vi "CVT2IndexReadTest.vi"() -> (3 "Unit Test Framework Results":T1)   [LabVIEW 2013, in "UnitTests.lvlib"]
uses:
  UnitTests.lvlib
  <vilib>/utf/common/utf_test_result_troll.ctl
  <vilib>/utf/common/utf_test_result.ctl
  <vilib>/utf/common/utf_test_result_failure.ctl
  <vilib>/utf/common/utf_test_comparison_operators.ctl
  <vilib>/utf/common/utf_vi_tag.ctl
  <vilib>/NI/Current Value Table/DataTypes/I32_Read Index.vi
  <vilib>/NI/Current Value Table/Memory Block.vi
  <vilib>/NI/Current Value Table/DataTypes/I32_Memory Block.vi
  <vilib>/utf/NI_UnitTestFramework.lvlib
  <vilib>/NI/Current Value Table/Current Value Table.lvlib
panel:
  out "Value":i32
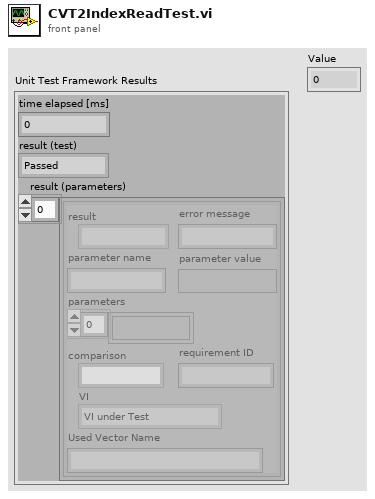
[diagram p1: front panel]
types:
  T1 = typedef "NI_UnitTestFramework.lvlib/utf_test_result_troll.ctl" = cluster{"time elapsed [ms]":u32, "result (test)":T2, "result (parameters)":T3[]}
  T2 = typedef "NI_UnitTestFramework.lvlib/utf_test_result.ctl" = enum16{"Passed", "Failed", "Error", "Skipped", "Not Processed"}
  T3 = typedef "NI_UnitTestFramework.lvlib/utf_test_result_failure.ctl" = cluster{"result":T2, "error message":string, "parameter name":string, "parameter value":variant, "parameters":variant[], "comparison":T4, "requirement ID":string, "VI":T5, "Used Vector Name":string}
  T4 = typedef "NI_UnitTestFramework.lvlib/utf_test_comparison_operators.ctl" = enum16{"=", "!=", ">", ">=", "<", "<=", "range", "symmetric tolerance", "asymmetric tolerance", "string contains", "string not contain", "array size", "string length", "array range", "by element", "array range (limit array)", "user-defined", "array contains", "array not contain", "vector length", "= (elm)", "!= (elm)", "= (case insensitive)", "!= (case insensitive)"}
  T5 = typedef "NI_UnitTestFramework.lvlib/utf_vi_tag.ctl" = enum16{"Setup VI", "VI under Test", "Teardown VI"}
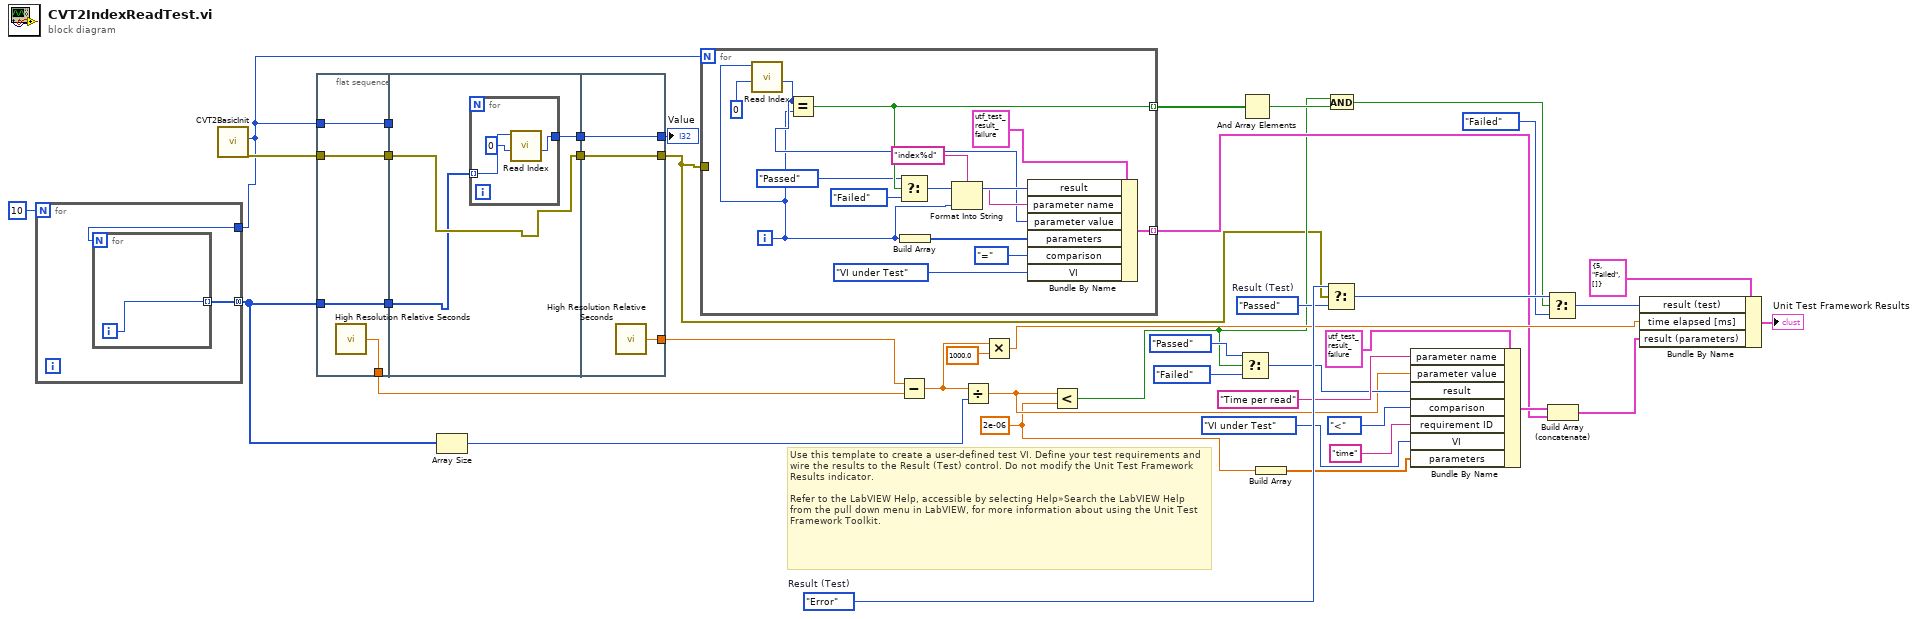
[diagram p0: block diagram]
diagram:
  w15 = 2e-06 ("y")
  w37 = utf_test_result."Error"  # Result (Test)
  w36 = utf_test_result."Passed"  # Result (Test)
  # "Use this template to create a user-defined test VI. Define your test requirements and wire the results to the Result (Test) control. Do not modify the Unit Test Framework Results indicator. \n\nRefer to the LabVIEW Help, accessible by selecting Help»Search the LabVIEW Help from the pull down menu in LabVIEW, for more information about using the Unit Test Framework Toolkit."
  n1 = call "CVT2BasicInit.vi"() -> ("error out"=w8:errorcluster, "Tags per type out"=w5:i32)  [unwired: 9 in, 1 out]
  n2 = for {
    N: 10 -> [_]
    tunnel: w5 -> [w44]
    tunnel: [w43] -> w3 mode=concatenating
    n3 = for {
      N: w44 -> [_]
      tunnel: [w45] -> w43 mode=indexing
      i -> [w45]
    }
  }
  n4 = flat-sequence {
    tunnel: [w49] -> w39
    tunnel: w8 -> [w47]
    tunnel: [w48] -> w31
    tunnel: w5 -> [w48]
    tunnel: [w47] -> w30
    tunnel: [w46] -> w4
    tunnel: w3 -> [w46]
    tunnel: w31 -> [_]
    tunnel: w30 -> [w51]
    tunnel: [w52] -> w10
    tunnel: [w51] -> w7
    tunnel: w4 -> [w50]
    tunnel: [w58] -> w40
    tunnel: [w57] -> w1
    tunnel: [w56] -> w9
    tunnel: w10 -> [w56]
    tunnel: w7 -> [w57]
    frame #0 {
      n5 = call <vilib>:"High Resolution Relative Seconds.vi"() -> ("relative seconds"=w49:dbl)
    }
    frame #1 {
      n6 = for {
        tunnel: [w54] -> w52
        tunnel: w50 -> [w53] mode=indexing
        n7 = call-poly <vilib>:"Read Index.vi"("Default"=0, "Index"=w53) -> ("Value"=w54:i32)  [unwired: 9 in]
      }
    }
    frame #2 {
      n8 = call <vilib>:"High Resolution Relative Seconds.vi"() -> ("relative seconds"=w58:dbl)
    }
  }
  n9 = Array Size(array=w3) -> (size(s)=w2:i32)
  n10 = for {
    N: w5 -> [_]
    tunnel: [w70] -> w27 mode=indexing
    tunnel: [w66] -> w13 mode=indexing
    tunnel: w1 -> [_]
    i -> [w59]
    n11 = call-poly <vilib>:"Read Index.vi"("Default"=0, "Index"=w59) -> ("Value"=w61:i32)  [unwired: 9 in]
    n12 = Equal?(x=w61, y=w59) -> (x = y?=w70:bool)
    n13 = Select(t=utf_test_result."Passed" ("result"), s=w70, f=utf_test_result."Failed" ("result")) -> (s? t:f=w67:T2)
    n14 = Build Array(w59) -> (w64:i32[])
    n15 = Format Into String(format string="index%d", w59) -> (resulting string=w63:string)  [unwired: 2 in, 1 out]
    n16 = Bundle By Name(cluster=T3 {"result"=enum."Passed", "error message"="", "parameter name"="", "parameter value"=variant, "parameters"=[], "comparison"=enum."=", "requirement ID"="", "VI"=enum."Setup VI", "Used Vector Name"=""} ("Unit Test Framework - result (parameters)"), "result"=w67, "parameter name"=w63, "parameter value"=w61, "parameters"=w64, "comparison"=utf_test_comparison_operators."=", "VI"=utf_vi_tag."VI under Test") -> (w66:T3)
  }
  n17 = Subtract(x=w40, y=w39) -> (x-y=w29:dbl)
  n18 = Divide(x=w29, y=w2) -> (x/y=w18:dbl)
  n19 = Multiply(x=w29, y=1000.0) -> (x*y=w32:dbl)
  n20 = Less?(x=w18, y=w15) -> (x < y?=w11:bool)
  n21 = Select(t=utf_test_result."Passed" ("result"), s=w11, f=utf_test_result."Failed" ("result")) -> (s? t:f=w19:T2)
  n22 = And Array Elements(Boolean array=w27) -> (logical AND=w26:bool)
  n23 = Build Array(w15) -> (w14:dbl[])
  n24 = Select(t=w37, s=w1, f=w36) -> (s? t:f=w25:T2)
  n25 = And(x=w11, y=w26) -> (x .and. y?=w12:bool)
  n26 = Bundle By Name(cluster=T3 {"result"=enum."Passed", "error message"="", "parameter name"="", "parameter value"=variant, "parameters"=[], "comparison"=enum."=", "requirement ID"="", "VI"=enum."Setup VI", "Used Vector Name"=""} ("Unit Test Framework - result (parameters)"), "parameter name"="Time per read", "parameter value"=w18, "result"=w19, "comparison"=utf_test_comparison_operators."<", "requirement ID"="time", "VI"=utf_vi_tag."VI under Test", "parameters"=w14) -> (w35:T3)
  n27 = Select(t=w25, s=w12, f=utf_test_result."Failed") -> (s? t:f=w23:T2)
  n28 = Build Array (concatenate)(w35, w13) -> (w34:T3[])
  n29 = Bundle By Name(cluster=T1 {"time elapsed [ms]"=5, "result (test)"=enum."Failed", "result (parameters)"=[]} ("Unit Test Framework - Result"), "result (test)"=w23, "time elapsed [ms]"=w32, "result (parameters)"=w34) -> (→"Unit Test Framework Results":T1)
  "Value" <- w9
